vi "Read EventsView.vi"(8 "error in (no error)":errorcluster, 11 "ProgrammaticInitialization in":refnum<class "ProgrammaticInitialization.lvclass">) -> (0 "error out":errorcluster, 2 "Events":T1, 3 "ProgrammaticInitialization out":refnum<class "ProgrammaticInitialization.lvclass">)   [LabVIEW 2016, in "ProgrammaticInitialization.lvclass"]
uses:
  ProgrammaticInitialization.lvclass
  evntsToSubscribeView.ctl
  ProgrammaticInitialization.lvclass/ProgrammaticInitialization.ctl
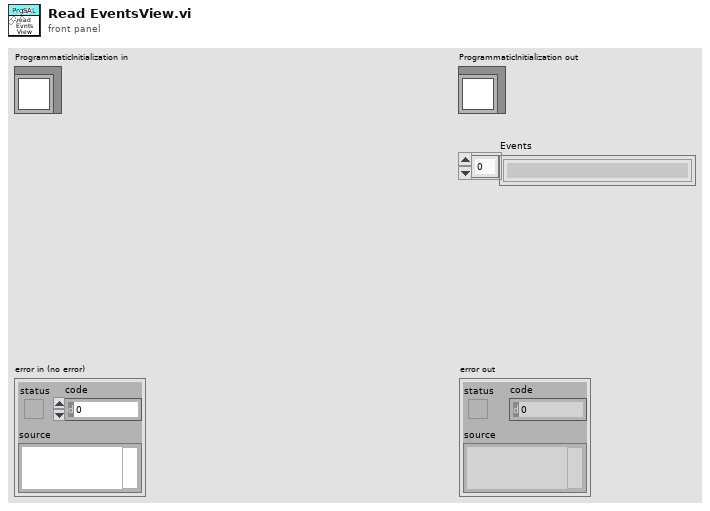
[diagram p1: front panel]
types:
  T1 = typedef "ProgrammaticInitialization.lvclass/evntsToSubscribeView.ctl" = string[]
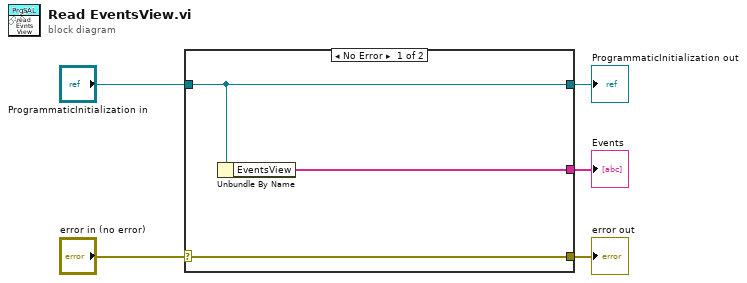
[diagram p0: block diagram]
diagram:
  n1 = case shown="No Error" "error in (no error)" {
    selector: "error in (no error)" -> [w8 w9]
    tunnel: [w8 w9] -> w4
    tunnel: [w7 w10] -> w2
    tunnel: "ProgrammaticInitialization in" -> [w7 w10]
    tunnel: [w6 _] -> w1
    frame No Error {
      n2 = Unbundle By Name(w7) -> ("EventsView"=w6:T1)
    }
    frame Error {
    }
  }
  "error out" <- w4
  "ProgrammaticInitialization out" <- w2
  "Events" <- w1
